vi "Freeze Value Array.vi"(0 "input array":dbl[](array[numeric]), 2 "Freeze Value":bool) -> (23 "output array":dbl[](array[numeric]))   [LabVIEW 2019, in "Untitled Library 1.lvlib"]
uses:
  Untitled Library 1.lvlib
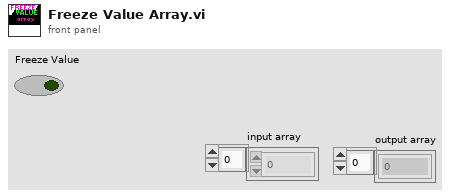
[diagram p1: front panel]
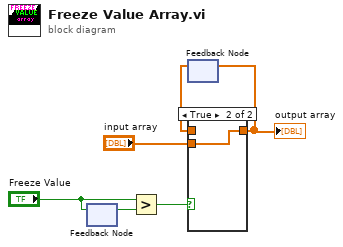
[diagram p0: block diagram]
diagram:
  n1 = feedback #1() -> (w6:bool)  [unwired: 1 in]
  n2 = feedback-in #1("Freeze Value") -> ()
  n3 = Greater?(x="Freeze Value", y=w6) -> (0:w4:bool)
  n4 = feedback #2() -> (w1:dbl[])  [unwired: 1 in]
  n5 = case shown="True" w4 {
    tunnel: "input array" -> [_ w8]
    tunnel: [w7 w8] -> w2
    tunnel: w1 -> [w7 _]
    frame False {
    }
    frame True {
    }
  }
  "output array" <- w2
  n6 = feedback-in #2(w2) -> ()
